vi "Trim Both Whitespace.vi"(0 "string":string) -> (2 "trimmed string":string)   [LabVIEW 2014, in "JKI State Machine++.lvlib"]
doc: "从 <B>string</B> 的开头、结尾或两者同时移除所有 ASCII 空白字符（空格、制表符、回车和换行）。\n\n<b>输入控件:</b>\n - <b>string</b>: 待处理字符串\n\n<b>输出控件:</b>\n - <b>trimmed string</b>: 处理后的字符串"
uses:
  JKI State Machine++.lvlib
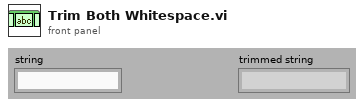
[diagram p1: front panel]
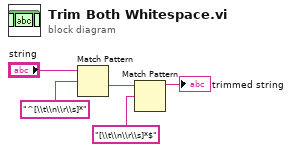
[diagram p0: block diagram]
diagram:
  n1 = Match Pattern(string="string", regular expression="^[\\t\\n\\r\\s]*") -> (after substring=w3:string)  [unwired: 1 in, 3 out]
  n2 = Match Pattern(string=w3, regular expression="[\\t\\n\\r\\s]*$") -> (before substring=→"trimmed string":string)  [unwired: 1 in, 3 out]
